vi "Counterforce.vi"(4 "ktrap":sgl, 6 "Ts":u32, 7 "alphacounterX":sgl, 8 "mobX(px/V)":sgl, 9 "SP_X":sgl, 10 "Xpx":sgl, 11 "Dx":sgl) -> (0 "Dts":sgl, 1 "ktrap*mob":sgl, 3 "counter Force":sgl)   [LabVIEW 2019]
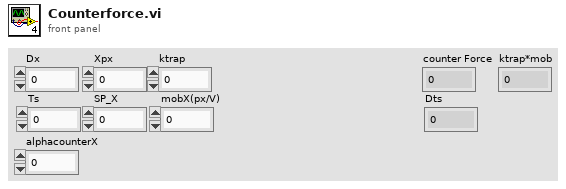
[diagram p1: front panel]
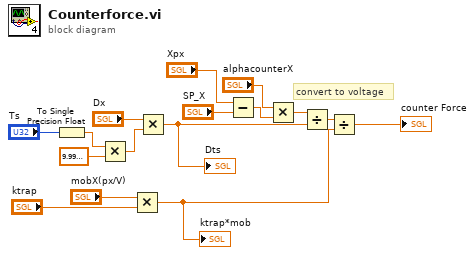
[diagram p0: block diagram]
diagram:
  # "convert to voltage"
  n1 = To Single Precision Float(number="Ts") -> (single precision float=w14:sgl)
  n2 = Multiply(x=w14, y=sgl 1e-06) -> (x*y=w12:sgl)
  n3 = Multiply(x="mobX(px/V)", y="ktrap") -> (x*y=w2:sgl)
  "ktrap*mob" <- w2
  n4 = Multiply(x="Dx", y=w12) -> (x*y=w5:sgl)
  "Dts" <- w5
  n5 = Subtract(x="Xpx", y="SP_X") -> (x-y=w9:sgl)
  n6 = Multiply(x="alphacounterX", y=w9) -> (x*y=w11:sgl)
  n7 = Divide(x=w11, y=w5) -> (x/y=w10:sgl)
  n8 = Divide(x=w10, y=w2) -> (x/y=→"counter Force":sgl)
